vi "Monitors_v00.vi"() -> ()   [LabVIEW 2011]
uses:
  <vilib>/measure/macond.llb/IIR Filter for N Chan.vi
  <vilib>/Analysis/5stat.llb/RMS (DBL).vi
  Global VIs/shotnoise.vi
  <vilib>/measure/NI_MAPro.lvlib
  <vilib>/Analysis/NI_AALPro.lvlib
  <vilib>/Analysis/NI_AALBase.lvlib
panel:
  in  "Shot noise start":bool
  out "Variance 1 normalised to SNL":dbl(graph)
  out "Variance 2 normalised to SNL":dbl(graph)
  out "conditional variance":dbl
  out "covariance":dbl
  in  "IIR filter specifications":T1={"Topology"=enum."Butterworth", "Type"=enum."Lowpass", "Order"=1, "Lower Fc"=100.0, "Upper Fc"=200.0, "PB Ripple"=1.0, "SB Attenuation"=60.0} {"PB Ripple" format="%0.2f"; "SB Attenuation" format="%0.2f"; "Lower Fc" format="%0.2p"; "Upper Fc" format="%0.2p"}
  in  "wfm":waveform(dbl)[](array[waveform])
  in  "error in":errorcluster caption="error out"
types:
  T1 = cluster{"Topology":enum16{"Off", "Butterworth", "Chebyshev", "Inverse Chebyshev", "Elliptic", "Bessel"}, "Type":enum16{"Lowpass", "Highpass", "Bandpass", "Bandstop"}, "Order":i32, "Lower Fc":dbl, "Upper Fc":dbl, "PB Ripple":dbl, "SB Attenuation":dbl}
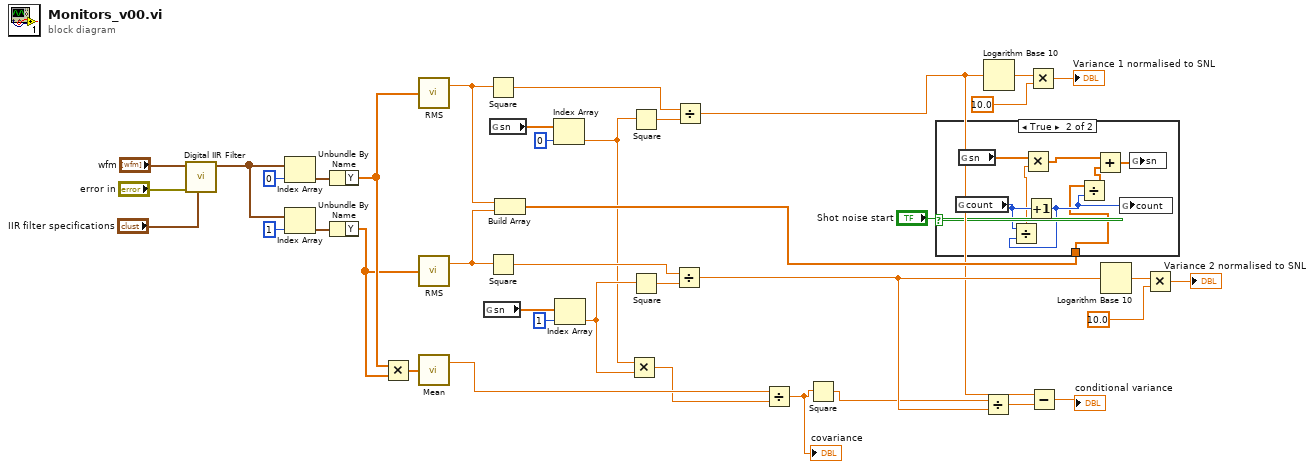
[diagram p0: block diagram]
diagram:
  n1 = call-poly <vilib>:"Digital IIR Filter.vi"("IIR filter specifications"="IIR filter specifications", "error in (no error)"="error in", "signal(s) in"="wfm") -> ("signal(s) out"=w1:waveform(dbl)[])  [unwired: 3 in, 5 out]
  n2 = Index Array(array=w1, index=0) -> (element=w13:waveform(dbl))
  n3 = Index Array(array=w1, index=1) -> (element=w18:waveform(dbl))
  n4 = Unbundle By Name(w13) -> ("Y"=w38:dbl[])
  n5 = Unbundle By Name(w18) -> ("Y"=w33:dbl[])
  n6 = Multiply(x=w38, y=w33) -> (x*y=w36:dbl[])
  n7 = call-poly <vilib>:"RMS.vi"("X"=w38) -> ("rms value"=w31:dbl)  [unwired: 1 out]
  n8 = call-poly <vilib>:"RMS.vi"("X"=w33) -> ("rms value"=w34:dbl)  [unwired: 1 out]
  n9 = call <vilib>:"Mean.vi"("X"=w36) -> ("mean"=w37:dbl)  [unwired: 1 out]
  n10 = global read "shotnoise.vi" "sn"() -> (w16:dbl[])
  n11 = Square(x=w31) -> (x^2=w32:dbl)
  n12 = Square(x=w34) -> (x^2=w35:dbl)
  n13 = global read "shotnoise.vi" "sn"() -> (w15:dbl[])
  n14 = Build Array(w31, w34) -> (w30:dbl[])
  n15 = Index Array(array=w15, index=0) -> (element=w26:dbl)
  n16 = Index Array(array=w16, index=1) -> (element=w27:dbl)
  n17 = Multiply(x=w26, y=w27) -> (x*y=w28:dbl)
  n18 = Square(x=w26) -> (x^2=w23:dbl)
  n19 = Square(x=w27) -> (x^2=w25:dbl)
  n20 = Divide(x=w35, y=w25) -> (x/y=w29:dbl)
  n21 = Divide(x=w32, y=w23) -> (x/y=w24:dbl)
  n22 = Divide(x=w37, y=w28) -> (x/y=w39:dbl)
  "covariance" <- w39
  n23 = Square(x=w39) -> (x^2=w20:dbl)
  n24 = case shown="True" "Shot noise start" {
    tunnel: w30 -> [_ w41]
    frame False {
    }
    frame True {
      n25 = global read "shotnoise.vi" "count"() -> (w46:i64)
      n26 = global read "shotnoise.vi" "sn"() -> (w45:dbl[])
      n27 = Increment(x=w46) -> (x+1=w42:i64)
      n28 = Divide(x=w46, y=w42) -> (x/y=w44:dbl)
      n29 = Multiply(x=w45, y=w44) -> (x*y=w43:dbl[])
      n30 = Divide(x=w41, y=w42) -> (x/y=w40:dbl[])
      n31 = Add(x=w43, y=w40) -> (x+y=w47:dbl[])
      n32 = global write "shotnoise.vi" "count"(w42) -> ()
      n33 = global write "shotnoise.vi" "sn"(w47) -> ()
    }
  }
  n34 = Divide(x=w20, y=w29) -> (x/y=w21:dbl)
  n35 = Logarithm Base 10(1:w24) -> (0:w5:dbl)
  n36 = Multiply(x=w5, y=10.0) -> (x*y=→"Variance 1 normalised to SNL":dbl)
  n37 = Subtract(x=w24, y=w21) -> (x-y=→"conditional variance":dbl)
  n38 = Logarithm Base 10(1:w29) -> (0:w8:dbl)
  n39 = Multiply(x=w8, y=10.0) -> (x*y=→"Variance 2 normalised to SNL":dbl)
